vi "水样测试.vi"(11 "数据标记表":string(combo)="N") -> ()   [LabVIEW 2016, in "斯坦道多参数.lvlib"]
panel:
  out "运行状态":u16(ring) items=["空闲", "水样测试", "标样核查"]
  out "多参数运行日志":string
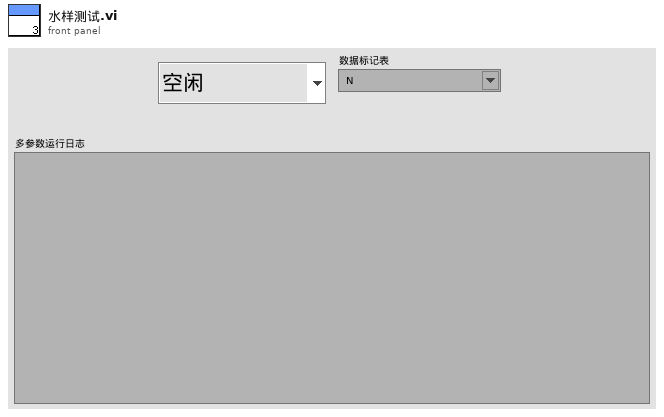
[diagram p1: front panel]
types:
  T1 = cluster{"水样数据时间":timestamp, "测量模式":string, "数据类型":string, "水样实测值":sgl, "单位":string, "水样数据标识":string, "信号值":sgl, "标样参考值":sgl, "因子编码":string, "探头温度":sgl}
  T2 = cluster{"水样数据时间":timestamp, "水温":dbl, "pH":dbl, "DO":dbl, "DOper":dbl, "电导率":dbl, "ORP":dbl, "浊度":dbl, "叶绿素a":dbl, "藻密度":dbl, "COD":dbl}
  T3 = cluster{"水温":bool, "pH":bool, "DO":bool, "DOper":bool, "电导率":bool, "ORP":bool, "浊度":bool, "叶绿素a":bool, "藻密度":bool, "COD":bool}
  T4 = cluster{"ph":bool, "DO":bool, "Cond":bool, "Turb":bool, "叶绿素a":bool, "藻密度":bool, "ORP":bool, "cod":bool}
  T5 = cluster{"温度测量值":sgl, "测量值":sgl, "温度偏移修正值":sgl, "信号值":sgl}
  T6 = cluster{"CH":u16, "监测值":dbl, "温度偏移修正值":sgl, "信号值":sgl}
  T7 = cluster{"温度测量值":sgl, "DO%":sgl, "DOmg/L":sgl, "温度偏移修正值":sgl}
  T8 = cluster{"测量量程":dbl, "测量精度":dbl, "测量间隔":dbl, "消解温度":dbl, "消解时长":dbl, "空白校准时间":timestamp, "曲线截距":dbl, "曲线斜率":dbl, "测量检出限":dbl, "测量信号值":dbl, "线性相关系数":dbl, "二次多项式系数":dbl, "标样校准时间":timestamp, "稀释倍数":dbl, "三项式系数":dbl, "空白标定系数":dbl, "量程系数":dbl, "F0/ORPA":dbl, "F1/ORPB":dbl, "F2/ORPK":dbl, "F3":dbl, "F4":dbl, "F5":dbl, "F6":dbl, "F7":dbl, "X0/滴定数":dbl, "量程":dbl}
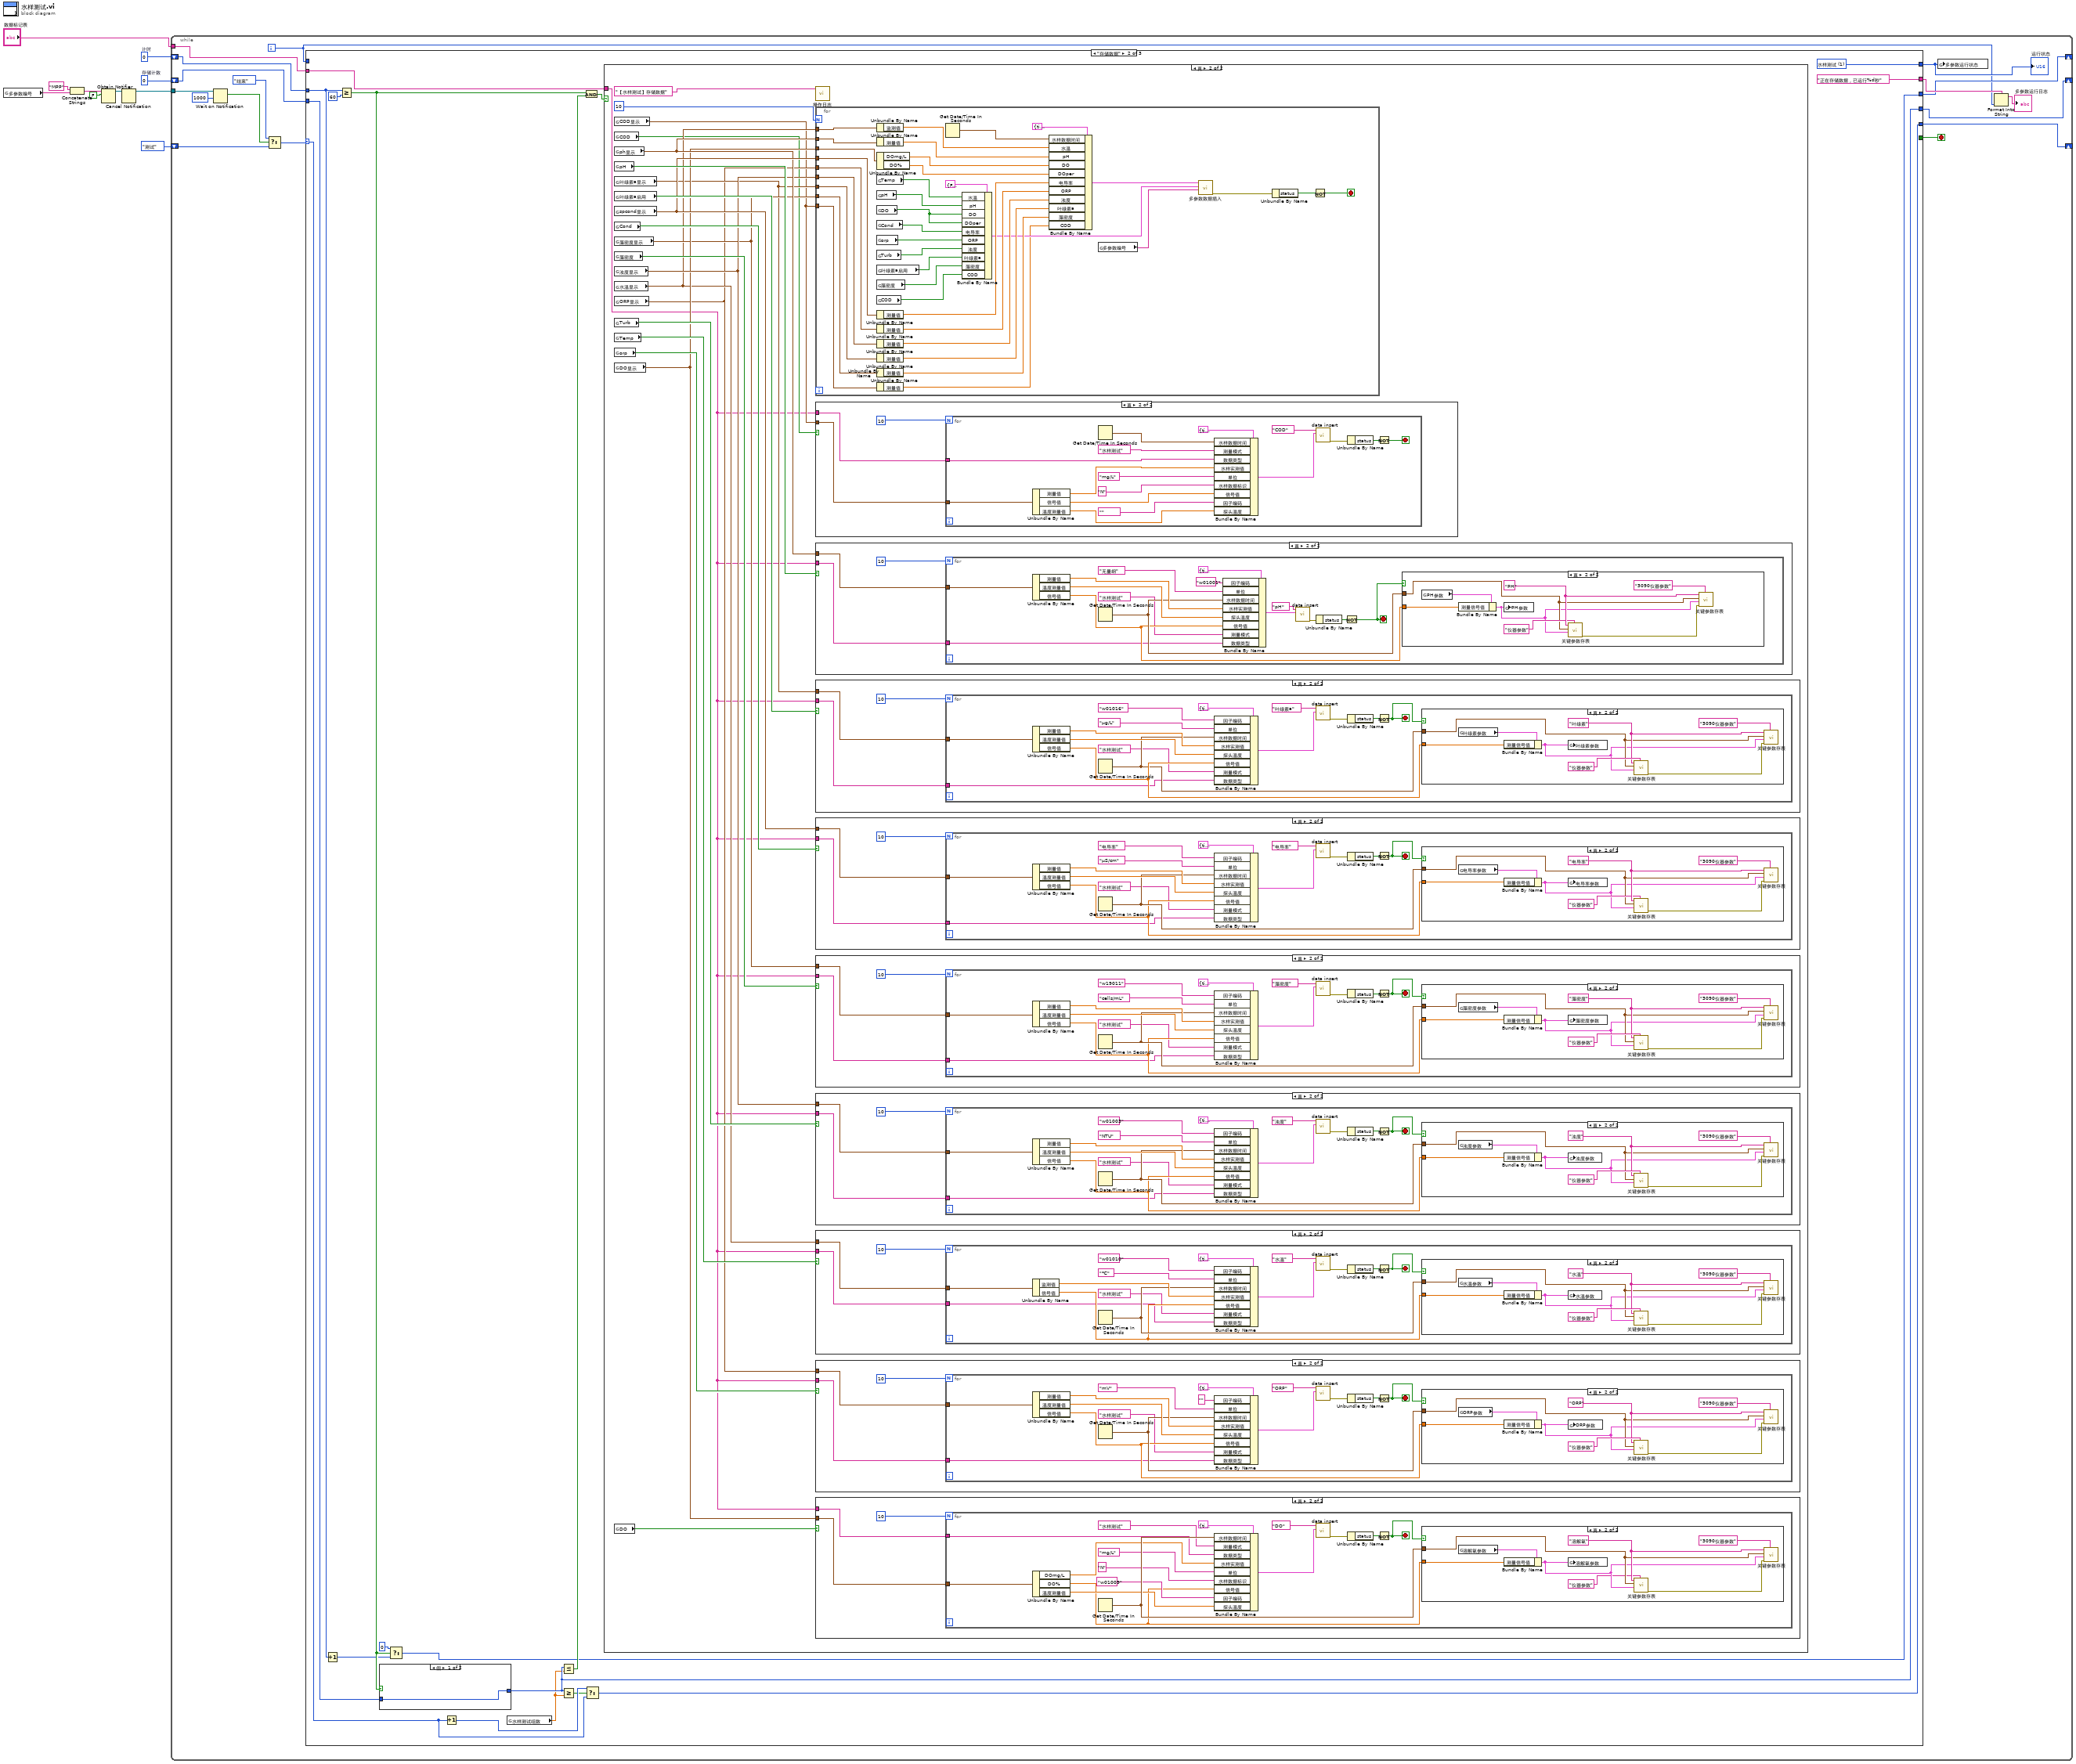
[diagram p0: block diagram]
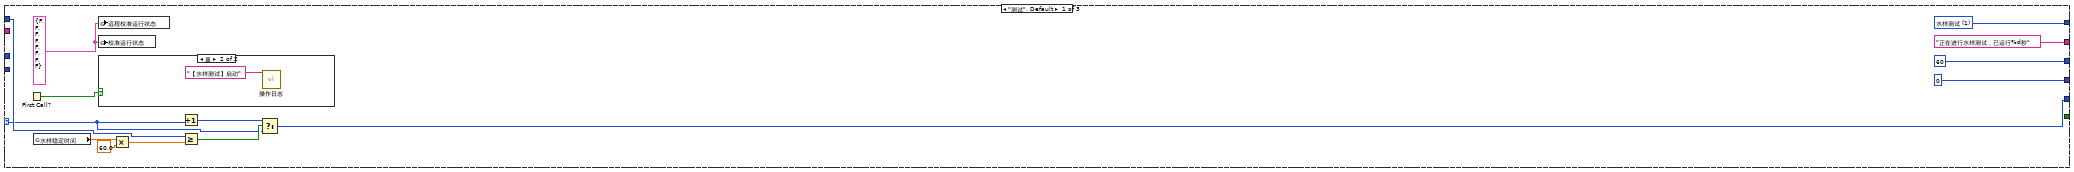
[diagram p2: hidden frame]
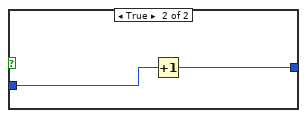
[diagram p4: hidden frame]
diagram:
  w1 = 0  # 存储计数
  w2 = 0  # 计时
  n1 = global read "多参数全局变量.vi" "多参数编号"() -> (w3:string)
  n2 = Concatenate Strings("MPP" ("名称（未命名）"), w3) -> (w4:string)
  n3 = Obtain Notifier(name (unnamed)=w4, notification data type=FALSE) -> (notifier out=w7:refnum<notifier>)  [unwired: 2 in, 2 out]
  n4 = Cancel Notification(0:w7) -> (8:w6:refnum<notifier>)  [unwired: 1 in, 2 out]
  n5 = while {
    shift-right: [w13] -> _
    shift-left: enum16{"测试", "存储数据", "结束"}."测试" ("枚举") -> [w11]
    tunnel: w6 -> [w24]
    tunnel: "数据标记表" -> [w19]
    shift-right: [w15] -> _
    shift-left: w2 -> [w17]
    shift-right: [w14] -> _
    shift-left: w1 -> [w16]
    i -> [w12]
    stop <- w27 stop-if-true
    n6 = Wait on Notification(notifier=w24, timeout in ms (-1)=1000 ("超时毫秒(-1)")) -> (notification=w22:bool)  [unwired: 2 in, 3 out]
    n7 = Select(t=enum16{"测试", "存储数据", "结束"}."结束" ("枚举"), s=w22, f=w11) -> (s? t:f=w20:enum16{"测试", "存储数据", "结束"})
    n8 = case shown="\"存储数据\"" w20 {
      selector: w20 -> [w33 w50 _]
      tunnel: [_ _ TRUE] -> w27
      tunnel: ["正在进行水样测试，已运行%d秒" ("格式字符串") "正在存储数据，已运行%d秒" ("格式字符串") "测试停止，累计运行%d秒" ("格式字符串")] -> w26
      tunnel: [w40 w55 w353] -> w18
      tunnel: w19 -> [_ w60 _]
      tunnel: w17 -> [_ w58 _]
      tunnel: w16 -> [_ w59 _]
      tunnel: [60 w43 0] -> w15
      tunnel: [0 w49 0] -> w14
      tunnel: [w31 w53 enum16{"测试", "存储数据", "结束"}."结束" ("枚举")] -> w13
      tunnel: w12 -> [w37 _ _]
      frame "测试", Default {
        w28 = T4 {"ph"=FALSE, "DO"=FALSE, "Cond"=FALSE, "Turb"=FALSE, "叶绿素a"=FALSE, "藻密度"=FALSE, "ORP"=FALSE, "cod"=FALSE} ("远程校准运行状态")
        w40 = u16 1 items=["空闲", "水样测试", "标样核查"] ("多参数运行状态")
        n9 = First Call?() -> (First Call?: T/F=w39:bool)
        n10 = global read "断电保存变量.vi" "水样稳定时间"() -> (w38:dbl)
        n11 = global write "多参数全局变量.vi" "远程校准运行状态"(w28) -> ()
        n12 = global write "多参数全局变量.vi" "校准运行状态"(w28) -> ()
        n13 = case shown="真" w39 {
          frame False {
          }
          frame True {
            n14 = call "操作日志.vi"("日志信息"="【水样测试】启动") -> ()  [unwired: 10 in, 1 out]
          }
        }
        n15 = Multiply(x=w38, y=60.0) -> (x*y=w35:dbl)
        n16 = Increment(x=w33) -> (x+1=w32:enum16{"测试", "存储数据", "结束"})
        n17 = Greater Or Equal?(x=w37, y=w35) -> (x >= y?=w34:bool)
        n18 = Select(t=w32, s=w34, f=w33) -> (s? t:f=w31:enum16{"测试", "存储数据", "结束"})
      }
      frame "存储数据" {
        w55 = u16 1 items=["空闲", "水样测试", "标样核查"] ("多参数运行状态")
        n19 = Increment(x=w58) -> (x+1=w45:i32)
        n20 = Greater Or Equal?(x=w58, y=60) -> (x >= y?=w46:bool)
        n21 = case shown="假" w46 {
          tunnel: w59 -> [w61 w63]
          tunnel: [w61 w62] -> w49
          frame False {
          }
          frame True {
            n22 = Increment(x=w63) -> (x+1=w62:i32)
          }
        }
        n23 = Select(t=0, s=w46, f=w45) -> (s? t:f=w43:i32)
        n24 = Increment(x=w50) -> (x+1=w51:enum16{"测试", "存储数据", "结束"})
        n25 = global read "断电保存变量.vi" "水样测试组数"() -> (w48:dbl)
        n26 = Less Or Equal?(x=w49, y=w48) -> (x <= y?=w54:bool)
        n27 = Greater Or Equal?(x=w49, y=w48) -> (x >= y?=w47:bool)
        n28 = And(x=w46, y=w54) -> (x .and. y?=w52:bool)
        n29 = Select(t=w51, s=w47, f=w50) -> (s? t:f=w53:enum16{"测试", "存储数据", "结束"})
        n30 = case shown="真" w52 {
          tunnel: w60 -> [_ w64]
          frame False {
          }
          frame True {
            n31 = global read "多参数全局变量.vi" "COD显示"() -> (w66:T5)
            n32 = global read "断电保存变量.vi" "COD"() -> (w65:bool)
            n33 = global read "多参数全局变量.vi" "ph显示"() -> (w74:T5)
            n34 = global read "断电保存变量.vi" "pH"() -> (w80:bool)
            n35 = global read "多参数全局变量.vi" "叶绿素a显示"() -> (w69:T5)
            n36 = global read "断电保存变量.vi" "叶绿素a启用"() -> (w84:bool)
            n37 = global read "多参数全局变量.vi" "spcond显示"() -> (w75:T5)
            n38 = global read "断电保存变量.vi" "Cond"() -> (w82:bool)
            n39 = global read "多参数全局变量.vi" "藻密度显示"() -> (w71:T5)
            n40 = global read "断电保存变量.vi" "藻密度"() -> (w78:bool)
            n41 = global read "多参数全局变量.vi" "浊度显示"() -> (w73:T5)
            n42 = global read "多参数全局变量.vi" "水温显示"() -> (w70:T6)
            n43 = global read "多参数全局变量.vi" "ORP显示"() -> (w68:T5)
            n44 = global read "断电保存变量.vi" "Turb"() -> (w83:bool)
            n45 = global read "断电保存变量.vi" "Temp"() -> (w79:bool)
            n46 = global read "断电保存变量.vi" "orp"() -> (w77:bool)
            n47 = global read "多参数全局变量.vi" "DO显示"() -> (w72:T7)
            n48 = global read "断电保存变量.vi" "DO"() -> (w81:bool)
            n49 = call "操作日志.vi"("日志信息"="【水样测试】存储数据") -> ()  [unwired: 10 in, 1 out]
            n50 = for {
              N: 10 -> [_]
              tunnel: w70 -> [w118]
              tunnel: w74 -> [w117]
              tunnel: w72 -> [w116]
              tunnel: w75 -> [w115]
              tunnel: w68 -> [w114]
              tunnel: w73 -> [w113]
              tunnel: w69 -> [w112]
              tunnel: w71 -> [w111]
              tunnel: w66 -> [w105]
              stop <- w120 stop-if-true
              n51 = Unbundle By Name(w118) -> ("监测值"=w139:dbl)
              n52 = Unbundle By Name(w117) -> ("测量值"=w138:sgl)
              n53 = Unbundle By Name(w116) -> ("DOmg/L"=w137:sgl, "DO%"=w136:sgl)
              n54 = global read "断电保存变量.vi" "Temp"() -> (w126:bool)
              n55 = global read "断电保存变量.vi" "pH"() -> (w130:bool)
              n56 = global read "断电保存变量.vi" "DO"() -> (w123:bool)
              n57 = global read "断电保存变量.vi" "Cond"() -> (w129:bool)
              n58 = global read "断电保存变量.vi" "orp"() -> (w125:bool)
              n59 = global read "断电保存变量.vi" "Turb"() -> (w128:bool)
              n60 = global read "断电保存变量.vi" "叶绿素a启用"() -> (w124:bool)
              n61 = global read "断电保存变量.vi" "藻密度"() -> (w127:bool)
              n62 = global read "断电保存变量.vi" "COD"() -> (w106:bool)
              n63 = Unbundle By Name(w115) -> ("测量值"=w135:sgl)
              n64 = Unbundle By Name(w114) -> ("测量值"=w134:sgl)
              n65 = Unbundle By Name(w113) -> ("测量值"=w133:sgl)
              n66 = Unbundle By Name(w112) -> ("测量值"=w131:sgl)
              n67 = Unbundle By Name(w111) -> ("测量值"=w132:sgl)
              n68 = Unbundle By Name(w105) -> ("测量值"=w104:sgl)
              n69 = Get Date/Time In Seconds() -> (seconds since 1Jan1904=w140:timestamp)
              n70 = Bundle By Name(cluster=T3 {"水温"=FALSE, "pH"=FALSE, "DO"=FALSE, "DOper"=FALSE, "电导率"=FALSE, "ORP"=FALSE, "浊度"=FALSE, "叶绿素a"=FALSE, "藻密度"=FALSE, "COD"=FALSE} ("columns enable"), "水温"=w126, "pH"=w130, "DO"=w123, "DOper"=w123, "电导率"=w129, "ORP"=w125, "浊度"=w128, "叶绿素a"=w124, "藻密度"=w127, "COD"=w106) -> (w107:T3)
              n71 = Bundle By Name(cluster=T2 {"水样数据时间"=timestamp(0 s since 1904-01-01), "水温"=0.0, "pH"=0.0, "DO"=0.0, "DOper"=0.0, "电导率"=0.0, "ORP"=0.0, "浊度"=0.0, "叶绿素a"=0.0, "藻密度"=0.0, "COD"=0.0} ("data in"), "水样数据时间"=w140, "水温"=w139, "pH"=w138, "DO"=w137, "DOper"=w136, "电导率"=w135, "ORP"=w134, "浊度"=w133, "叶绿素a"=w131, "藻密度"=w132, "COD"=w104) -> (w108:T2)
              n72 = global read "多参数全局变量.vi" "多参数编号"() -> (w119:string)
              n73 = call "多参数数据插入.vi"("编号"=w119, "columns enable"=w107, "data in"=w108) -> ("error out"=w122:errorcluster)  [unwired: 8 in]
              n74 = Unbundle By Name(w122) -> ("status"=w121:bool)
              n75 = Not(x=w121) -> (.not. x?=w120:bool)
            }
            n76 = case shown="真" w65 {
              tunnel: w64 -> [_ w87]
              tunnel: w66 -> [_ w85]
              frame False {
              }
              frame True {
                n77 = for {
                  N: 10 -> [_]
                  tunnel: w87 -> [w99]
                  tunnel: w85 -> [w88]
                  stop <- w103 stop-if-true
                  n78 = Unbundle By Name(w88) -> ("测量值"=w98:sgl, "信号值"=w91:sgl, "温度测量值"=w92:sgl)
                  n79 = Get Date/Time In Seconds() -> (seconds since 1Jan1904=w101:timestamp)
                  n80 = Bundle By Name(cluster=T1 {"水样数据时间"=timestamp(0 s since 1904-01-01), "测量模式"="", "数据类型"="N", "水样实测值"=0.0, "单位"="", "水样数据标识"="N", "信号值"=0.0, "标样参考值"=0.0, "因子编码"="", "探头温度"=0.0} ("data in"), "水样数据时间"=w101, "测量模式"="水样测试", "数据类型"=w99, "水样实测值"=w98, "单位"="mg/L", "水样数据标识"="N", "信号值"=w91, "因子编码"="", "探头温度"=w92) -> (w89:T1)
                  n81 = call "data insert.vi"("data in"=w89, "table in"="COD") -> ("error out"=w94:errorcluster)  [unwired: 9 in]
                  n82 = Unbundle By Name(w94) -> ("status"=w95:bool)
                  n83 = Not(x=w95) -> (.not. x?=w103:bool)
                }
              }
            }
            n84 = case shown="真" w80 {
              tunnel: w64 -> [_ w300]
              tunnel: w74 -> [_ w298]
              frame False {
              }
              frame True {
                n85 = for {
                  N: 10 -> [_]
                  tunnel: w300 -> [w302]
                  tunnel: w298 -> [w301]
                  stop <- w307 stop-if-true
                  n86 = Unbundle By Name(w301) -> ("测量值"=w311:sgl, "温度测量值"=w310:sgl, "信号值"=w305:sgl)
                  n87 = Get Date/Time In Seconds() -> (seconds since 1Jan1904=w306:timestamp)
                  n88 = Bundle By Name(cluster=T1 {"水样数据时间"=timestamp(0 s since 1904-01-01), "测量模式"="", "数据类型"="N", "水样实测值"=0.0, "单位"="", "水样数据标识"="N", "信号值"=0.0, "标样参考值"=0.0, "因子编码"="", "探头温度"=0.0} ("data in"), "因子编码"="w01001", "单位"="无量纲", "水样数据时间"=w306, "水样实测值"=w311, "探头温度"=w310, "信号值"=w305, "测量模式"="水样测试", "数据类型"=w302) -> (w315:T1)
                  n89 = call "data insert.vi"("data in"=w315, "table in"="pH" ("table输入")) -> ("error out"=w309:errorcluster)  [unwired: 9 in]
                  n90 = Unbundle By Name(w309) -> ("status"=w308:bool)
                  n91 = Not(x=w308) -> (.not. x?=w307:bool)
                  n92 = case shown="真" w307 {
                    tunnel: w306 -> [_ w318]
                    tunnel: w305 -> [_ w322]
                    frame False {
                    }
                    frame True {
                      w321 = "PH" ("仪器名称")
                      n93 = global read "断电保存变量.vi" "PH参数"() -> (w323:T8)
                      n94 = Bundle By Name(cluster=w323, "测量信号值"=w322) -> (w317:T8)
                      n95 = global write "断电保存变量.vi" "PH参数"(w317) -> ()
                      n96 = call "关键参数存表.vi"("table"="仪器参数", "仪器参数"=w317, "datatime"=w318, "仪器名称"=w321) -> ("error out"=w316:errorcluster)  [unwired: 7 in]
                      n97 = call "关键参数存表.vi"("table"="3090仪器参数", "error in (no error)"=w316, "仪器参数"=w317, "datatime"=w318, "仪器名称"=w321) -> ()  [unwired: 6 in, 1 out]
                    }
                  }
                }
              }
            }
            n98 = case shown="真" w84 {
              tunnel: w64 -> [_ w195]
              tunnel: w69 -> [_ w193]
              frame False {
              }
              frame True {
                n99 = for {
                  N: 10 -> [_]
                  tunnel: w195 -> [w197]
                  tunnel: w193 -> [w196]
                  stop <- w202 stop-if-true
                  n100 = Unbundle By Name(w196) -> ("测量值"=w210:sgl, "温度测量值"=w209:sgl, "信号值"=w201:sgl)
                  n101 = Get Date/Time In Seconds() -> (seconds since 1Jan1904=w200:timestamp)
                  n102 = Bundle By Name(cluster=T1 {"水样数据时间"=timestamp(0 s since 1904-01-01), "测量模式"="", "数据类型"="N", "水样实测值"=0.0, "单位"="", "水样数据标识"="N", "信号值"=0.0, "标样参考值"=0.0, "因子编码"="", "探头温度"=0.0} ("data in"), "因子编码"="w01016", "单位"="μg/L", "水样数据时间"=w200, "水样实测值"=w210, "探头温度"=w209, "信号值"=w201, "测量模式"="水样测试", "数据类型"=w197) -> (w207:T1)
                  n103 = call "data insert.vi"("data in"=w207, "table in"="叶绿素a" ("table输入")) -> ("error out"=w205:errorcluster)  [unwired: 9 in]
                  n104 = Unbundle By Name(w205) -> ("status"=w204:bool)
                  n105 = Not(x=w204) -> (.not. x?=w202:bool)
                  n106 = case shown="真" w202 {
                    tunnel: w200 -> [_ w213]
                    tunnel: w201 -> [_ w217]
                    frame False {
                    }
                    frame True {
                      w214 = "叶绿素" ("仪器名称")
                      n107 = global read "断电保存变量.vi" "叶绿素参数"() -> (w218:T8)
                      n108 = Bundle By Name(cluster=w218, "测量信号值"=w217) -> (w212:T8)
                      n109 = global write "断电保存变量.vi" "叶绿素参数"(w212) -> ()
                      n110 = call "关键参数存表.vi"("table"="仪器参数", "仪器参数"=w212, "datatime"=w213, "仪器名称"=w214) -> ("error out"=w211:errorcluster)  [unwired: 7 in]
                      n111 = call "关键参数存表.vi"("table"="3090仪器参数", "error in (no error)"=w211, "仪器参数"=w212, "datatime"=w213, "仪器名称"=w214) -> ()  [unwired: 6 in, 1 out]
                    }
                  }
                }
              }
            }
            n112 = case shown="真" w82 {
              tunnel: w64 -> [_ w247]
              tunnel: w75 -> [_ w245]
              frame False {
              }
              frame True {
                n113 = for {
                  N: 10 -> [_]
                  tunnel: w247 -> [w249]
                  tunnel: w245 -> [w248]
                  stop <- w255 stop-if-true
                  n114 = Unbundle By Name(w248) -> ("测量值"=w260:sgl, "温度测量值"=w259:sgl, "信号值"=w253:sgl)
                  n115 = Get Date/Time In Seconds() -> (seconds since 1Jan1904=w254:timestamp)
                  n116 = Bundle By Name(cluster=T1 {"水样数据时间"=timestamp(0 s since 1904-01-01), "测量模式"="", "数据类型"="N", "水样实测值"=0.0, "单位"="", "水样数据标识"="N", "信号值"=0.0, "标样参考值"=0.0, "因子编码"="", "探头温度"=0.0} ("data in"), "因子编码"="电导率", "单位"="μS/cm", "水样数据时间"=w254, "水样实测值"=w260, "探头温度"=w259, "信号值"=w253, "测量模式"="水样测试", "数据类型"=w249) -> (w250:T1)
                  n117 = call "data insert.vi"("data in"=w250, "table in"="电导率" ("table输入")) -> ("error out"=w258:errorcluster)  [unwired: 9 in]
                  n118 = Unbundle By Name(w258) -> ("status"=w257:bool)
                  n119 = Not(x=w257) -> (.not. x?=w255:bool)
                  n120 = case shown="真" w255 {
                    tunnel: w254 -> [_ w265]
                    tunnel: w253 -> [_ w269]
                    frame False {
                    }
                    frame True {
                      w268 = "电导率" ("仪器名称")
                      n121 = global read "断电保存变量.vi" "电导率参数"() -> (w270:T8)
                      n122 = Bundle By Name(cluster=w270, "测量信号值"=w269) -> (w264:T8)
                      n123 = global write "断电保存变量.vi" "电导率参数"(w264) -> ()
                      n124 = call "关键参数存表.vi"("table"="仪器参数", "仪器参数"=w264, "datatime"=w265, "仪器名称"=w268) -> ("error out"=w263:errorcluster)  [unwired: 7 in]
                      n125 = call "关键参数存表.vi"("table"="3090仪器参数", "error in (no error)"=w263, "仪器参数"=w264, "datatime"=w265, "仪器名称"=w268) -> ()  [unwired: 6 in, 1 out]
                    }
                  }
                }
              }
            }
            n126 = case shown="真" w78 {
              tunnel: w64 -> [_ w169]
              tunnel: w71 -> [_ w167]
              frame False {
              }
              frame True {
                n127 = for {
                  N: 10 -> [_]
                  tunnel: w169 -> [w172]
                  tunnel: w167 -> [w170]
                  stop <- w174 stop-if-true
                  n128 = Unbundle By Name(w170) -> ("测量值"=w184:sgl, "温度测量值"=w182:sgl, "信号值"=w175:sgl)
                  n129 = Get Date/Time In Seconds() -> (seconds since 1Jan1904=w176:timestamp)
                  n130 = Bundle By Name(cluster=T1 {"水样数据时间"=timestamp(0 s since 1904-01-01), "测量模式"="", "数据类型"="N", "水样实测值"=0.0, "单位"="", "水样数据标识"="N", "信号值"=0.0, "标样参考值"=0.0, "因子编码"="", "探头温度"=0.0} ("data in"), "因子编码"="w19011", "单位"="cells/mL", "水样数据时间"=w176, "水样实测值"=w184, "探头温度"=w182, "信号值"=w175, "测量模式"="水样测试", "数据类型"=w172) -> (w177:T1)
                  n131 = call "data insert.vi"("data in"=w177, "table in"="藻密度" ("table输入")) -> ("error out"=w179:errorcluster)  [unwired: 9 in]
                  n132 = Unbundle By Name(w179) -> ("status"=w178:bool)
                  n133 = Not(x=w178) -> (.not. x?=w174:bool)
                  n134 = case shown="真" w174 {
                    tunnel: w176 -> [_ w188]
                    tunnel: w175 -> [_ w191]
                    frame False {
                    }
                    frame True {
                      w189 = "藻密度" ("仪器名称")
                      n135 = global read "断电保存变量.vi" "藻密度参数"() -> (w192:T8)
                      n136 = Bundle By Name(cluster=w192, "测量信号值"=w191) -> (w187:T8)
                      n137 = global write "断电保存变量.vi" "藻密度参数"(w187) -> ()
                      n138 = call "关键参数存表.vi"("table"="仪器参数", "仪器参数"=w187, "datatime"=w188, "仪器名称"=w189) -> ("error out"=w186:errorcluster)  [unwired: 7 in]
                      n139 = call "关键参数存表.vi"("table"="3090仪器参数", "error in (no error)"=w186, "仪器参数"=w187, "datatime"=w188, "仪器名称"=w189) -> ()  [unwired: 6 in, 1 out]
                    }
                  }
                }
              }
            }
            n140 = case shown="真" w83 {
              tunnel: w64 -> [_ w221]
              tunnel: w73 -> [_ w219]
              frame False {
              }
              frame True {
                n141 = for {
                  N: 10 -> [_]
                  tunnel: w221 -> [w223]
                  tunnel: w219 -> [w222]
                  stop <- w228 stop-if-true
                  n142 = Unbundle By Name(w222) -> ("测量值"=w232:sgl, "温度测量值"=w231:sgl, "信号值"=w226:sgl)
                  n143 = Get Date/Time In Seconds() -> (seconds since 1Jan1904=w227:timestamp)
                  n144 = Bundle By Name(cluster=T1 {"水样数据时间"=timestamp(0 s since 1904-01-01), "测量模式"="", "数据类型"="N", "水样实测值"=0.0, "单位"="", "水样数据标识"="N", "信号值"=0.0, "标样参考值"=0.0, "因子编码"="", "探头温度"=0.0} ("data in"), "因子编码"="w01003", "单位"="NTU", "水样数据时间"=w227, "水样实测值"=w232, "探头温度"=w231, "信号值"=w226, "测量模式"="水样测试", "数据类型"=w223) -> (w235:T1)
                  n145 = call "data insert.vi"("data in"=w235, "table in"="浊度" ("table输入")) -> ("error out"=w230:errorcluster)  [unwired: 9 in]
                  n146 = Unbundle By Name(w230) -> ("status"=w229:bool)
                  n147 = Not(x=w229) -> (.not. x?=w228:bool)
                  n148 = case shown="真" w228 {
                    tunnel: w227 -> [_ w239]
                    tunnel: w226 -> [_ w243]
                    frame False {
                    }
                    frame True {
                      w240 = "浊度" ("仪器名称")
                      n149 = global read "断电保存变量.vi" "浊度参数"() -> (w244:T8)
                      n150 = Bundle By Name(cluster=w244, "测量信号值"=w243) -> (w238:T8)
                      n151 = global write "断电保存变量.vi" "浊度参数"(w238) -> ()
                      n152 = call "关键参数存表.vi"("table"="仪器参数", "仪器参数"=w238, "datatime"=w239, "仪器名称"=w240) -> ("error out"=w237:errorcluster)  [unwired: 7 in]
                      n153 = call "关键参数存表.vi"("table"="3090仪器参数", "error in (no error)"=w237, "仪器参数"=w238, "datatime"=w239, "仪器名称"=w240) -> ()  [unwired: 6 in, 1 out]
                    }
                  }
                }
              }
            }
            n154 = case shown="真" w79 {
              tunnel: w64 -> [_ w326]
              tunnel: w70 -> [_ w324]
              frame False {
              }
              frame True {
                n155 = for {
                  N: 10 -> [_]
                  tunnel: w326 -> [w328]
                  tunnel: w324 -> [w327]
                  stop <- w333 stop-if-true
                  n156 = Unbundle By Name(w327) -> ("监测值"=w336:dbl, "信号值"=w331:sgl)
                  n157 = Get Date/Time In Seconds() -> (seconds since 1Jan1904=w332:timestamp)
                  n158 = Bundle By Name(cluster=T1 {"水样数据时间"=timestamp(0 s since 1904-01-01), "测量模式"="", "数据类型"="N", "水样实测值"=0.0, "单位"="", "水样数据标识"="N", "信号值"=0.0, "标样参考值"=0.0, "因子编码"="", "探头温度"=0.0} ("data in"), "因子编码"="w01010", "单位"="℃", "水样数据时间"=w332, "水样实测值"=w336, "信号值"=w331, "测量模式"="水样测试", "数据类型"=w328) -> (w339:T1)
                  n159 = call "data insert.vi"("data in"=w339, "table in"="水温" ("table输入")) -> ("error out"=w335:errorcluster)  [unwired: 9 in]
                  n160 = Unbundle By Name(w335) -> ("status"=w334:bool)
                  n161 = Not(x=w334) -> (.not. x?=w333:bool)
                  n162 = case shown="真" w333 {
                    tunnel: w332 -> [_ w344]
                    tunnel: w331 -> [_ w347]
                    frame False {
                    }
                    frame True {
                      w345 = "水温" ("仪器名称")
                      n163 = global read "断电保存变量.vi" "水温参数"() -> (w348:T8)
                      n164 = Bundle By Name(cluster=w348, "测量信号值"=w347) -> (w343:T8)
                      n165 = global write "断电保存变量.vi" "水温参数"(w343) -> ()
                      n166 = call "关键参数存表.vi"("table"="仪器参数", "仪器参数"=w343, "datatime"=w344, "仪器名称"=w345) -> ("error out"=w342:errorcluster)  [unwired: 7 in]
                      n167 = call "关键参数存表.vi"("table"="3090仪器参数", "error in (no error)"=w342, "仪器参数"=w343, "datatime"=w344, "仪器名称"=w345) -> ()  [unwired: 6 in, 1 out]
                    }
                  }
                }
              }
            }
            n168 = case shown="真" w77 {
              tunnel: w64 -> [_ w143]
              tunnel: w68 -> [_ w141]
              frame False {
              }
              frame True {
                n169 = for {
                  N: 10 -> [_]
                  tunnel: w143 -> [w146]
                  tunnel: w141 -> [w144]
                  stop <- w151 stop-if-true
                  n170 = Unbundle By Name(w144) -> ("测量值"=w158:sgl, "温度测量值"=w156:sgl, "信号值"=w149:sgl)
                  n171 = Get Date/Time In Seconds() -> (seconds since 1Jan1904=w150:timestamp)
                  n172 = Bundle By Name(cluster=T1 {"水样数据时间"=timestamp(0 s since 1904-01-01), "测量模式"="", "数据类型"="N", "水样实测值"=0.0, "单位"="", "水样数据标识"="N", "信号值"=0.0, "标样参考值"=0.0, "因子编码"="", "探头温度"=0.0} ("data in"), "因子编码"="", "单位"="mV", "水样数据时间"=w150, "水样实测值"=w158, "探头温度"=w156, "信号值"=w149, "测量模式"="水样测试", "数据类型"=w146) -> (w147:T1)
                  n173 = call "data insert.vi"("data in"=w147, "table in"="ORP" ("table输入")) -> ("error out"=w154:errorcluster)  [unwired: 9 in]
                  n174 = Unbundle By Name(w154) -> ("status"=w153:bool)
                  n175 = Not(x=w153) -> (.not. x?=w151:bool)
                  n176 = case shown="真" w151 {
                    tunnel: w150 -> [_ w162]
                    tunnel: w149 -> [_ w165]
                    frame False {
                    }
                    frame True {
                      w163 = "ORP" ("仪器名称")
                      n177 = global read "断电保存变量.vi" "ORP参数"() -> (w166:T8)
                      n178 = Bundle By Name(cluster=w166, "测量信号值"=w165) -> (w161:T8)
                      n179 = global write "断电保存变量.vi" "ORP参数"(w161) -> ()
                      n180 = call "关键参数存表.vi"("table"="仪器参数", "仪器参数"=w161, "datatime"=w162, "仪器名称"=w163) -> ("error out"=w160:errorcluster)  [unwired: 7 in]
                      n181 = call "关键参数存表.vi"("table"="3090仪器参数", "error in (no error)"=w160, "仪器参数"=w161, "datatime"=w162, "仪器名称"=w163) -> ()  [unwired: 6 in, 1 out]
                    }
                  }
                }
              }
            }
            n182 = case shown="真" w81 {
              tunnel: w64 -> [_ w273]
              tunnel: w72 -> [_ w271]
              frame False {
              }
              frame True {
                n183 = for {
                  N: 10 -> [_]
                  tunnel: w273 -> [w285]
                  tunnel: w271 -> [w274]
                  stop <- w289 stop-if-true
                  n184 = Unbundle By Name(w274) -> ("DOmg/L"=w284:sgl, "DO%"=w277:sgl, "温度测量值"=w278:sgl)
                  n185 = Get Date/Time In Seconds() -> (seconds since 1Jan1904=w287:timestamp)
                  n186 = Bundle By Name(cluster=T1 {"水样数据时间"=timestamp(0 s since 1904-01-01), "测量模式"="", "数据类型"="N", "水样实测值"=0.0, "单位"="", "水样数据标识"="N", "信号值"=0.0, "标样参考值"=0.0, "因子编码"="", "探头温度"=0.0} ("data in"), "水样数据时间"=w287, "测量模式"="水样测试", "数据类型"=w285, "水样实测值"=w284, "单位"="mg/L", "水样数据标识"="N", "信号值"=w277, "因子编码"="w01009", "探头温度"=w278) -> (w275:T1)
                  n187 = call "data insert.vi"("data in"=w275, "table in"="DO") -> ("error out"=w280:errorcluster)  [unwired: 9 in]
                  n188 = Unbundle By Name(w280) -> ("status"=w281:bool)
                  n189 = Not(x=w281) -> (.not. x?=w289:bool)
                  n190 = case shown="真" w289 {
                    tunnel: w287 -> [_ w294]
                    tunnel: w277 -> [_ w296]
                    frame False {
                    }
                    frame True {
                      w295 = "溶解氧" ("仪器名称")
                      n191 = global read "断电保存变量.vi" "溶解氧参数"() -> (w297:T8)
                      n192 = Bundle By Name(cluster=w297, "测量信号值"=w296) -> (w293:T8)
                      n193 = global write "断电保存变量.vi" "溶解氧参数"(w293) -> ()
                      n194 = call "关键参数存表.vi"("table"="仪器参数", "仪器参数"=w293, "datatime"=w294, "仪器名称"=w295) -> ("error out"=w292:errorcluster)  [unwired: 7 in]
                      n195 = call "关键参数存表.vi"("table"="3090仪器参数", "error in (no error)"=w292, "仪器参数"=w293, "datatime"=w294, "仪器名称"=w295) -> ()  [unwired: 6 in, 1 out]
                    }
                  }
                }
              }
            }
          }
        }
      }
      frame "结束" {
        w353 = u16 0 items=["空闲", "水样测试", "标样核查"] ("多参数运行状态")
        n196 = First Call?() -> (First Call?: T/F=w352:bool)
        n197 = case shown="真" w352 {
          frame False {
          }
          frame True {
            n198 = call "操作日志.vi"("日志信息"="【水样测试】结束") -> ()  [unwired: 10 in, 1 out]
          }
        }
      }
    }
    "运行状态" <- w18
    n199 = global write "多参数全局变量.vi" "多参数运行状态"(w18) -> ()
    n200 = Format Into String(format string=w26, w12) -> (resulting string=→"多参数运行日志":string)  [unwired: 2 in, 1 out]
  }
